vi "WriteToFile-v1.vi"(5 "Array":string[](array[string]), 7 "String":string, 8 "error in (no error)":errorcluster, 9 "rt fifo":refnum<k33>, 10 "Boolean":bool, 11 "Refnum in":refnum<k34>) -> (0 "error out 2":errorcluster, 2 "Writing?":bool=TRUE, 3 "Refnum out":refnum<k34>)   [LabVIEW 2018]
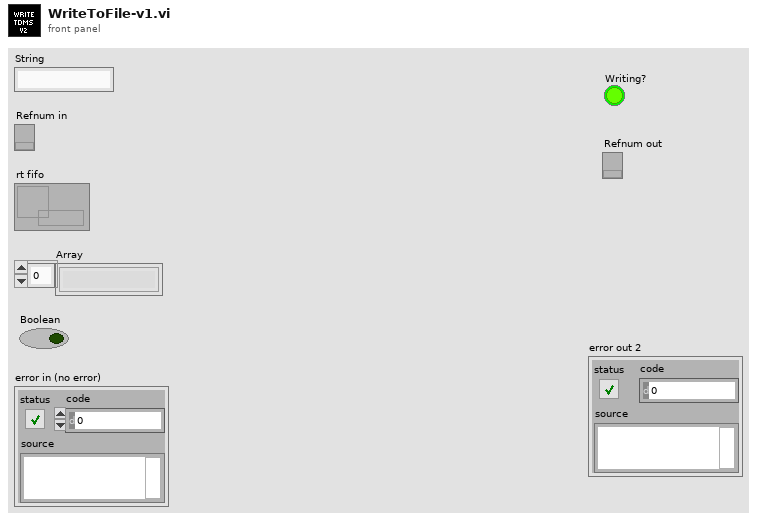
[diagram p1: front panel]
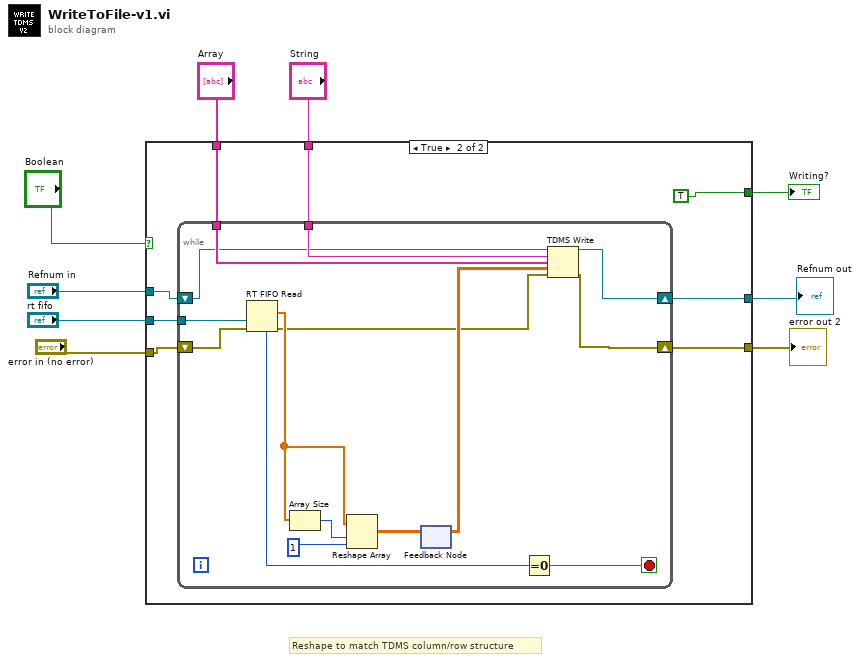
[diagram p0: block diagram]
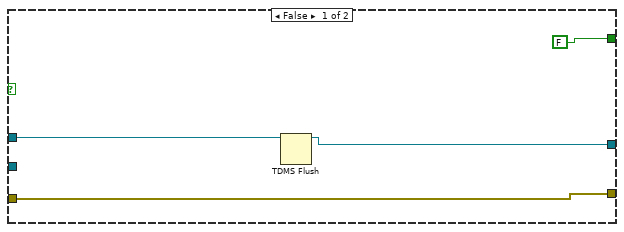
[diagram p2: hidden frame]
diagram:
  # "Reshape to match TDMS column/row structure"
  n1 = case shown="True" "Boolean" {
    tunnel: "String" -> [_ w21]
    tunnel: "Array" -> [_ w20]
    tunnel: [w11 w19] -> w7
    tunnel: [w12 w18] -> w6
    tunnel: "error in (no error)" -> [w11 w17]
    tunnel: "rt fifo" -> [_ w16]
    tunnel: "Refnum in" -> [w13 w15]
    tunnel: [FALSE TRUE] -> w1
    frame False {
      n2 = TDMS Flush(7:w13) -> (3:w12:refnum<k34>)  [unwired: 1 in, 1 out]
    }
    frame True {
      n3 = while {
        tunnel: w21 -> [w35]
        tunnel: w20 -> [w34]
        tunnel: w16 -> [w25]
        shift-right: [w28] -> w19
        shift-left: w17 -> [w26]
        shift-right: [w27] -> w18
        shift-left: w15 -> [w24]
        stop <- w22 stop-if-true
        n4 = RT FIFO Read(0:w25, 3:w26) -> (7:w23:u32, 9:w31:dbl[], 11:w29:errorcluster)  [unwired: 2 in, 2 out]
        n5 = Array Size(array=w31) -> (size(s)=w36:i32)
        n6 = Reshape Array(w31, w36, 1) -> (w32:dbl[][])
        n7 = feedback #1() -> (w33:dbl[][])  [unwired: 1 in]
        n8 = feedback-in #1(w32) -> ()
        n9 = Equal To 0?(x=w23) -> (x = 0?=w22:bool)
        n10 = TDMS Write(0:w24, 5:w35, 7:w34, 9:w33, 11:w29) -> (4:w27:refnum<k34>, 15:w28:errorcluster)  [unwired: 1 in, 2 out]
      }
    }
  }
  "Refnum out" <- w6
  "error out 2" <- w7
  "Writing?" <- w1
